vi "Tom_Bentham_New_FF.vi"() -> (5 "Plug in titles":string[](array[string]), 7 "Plug in values":string[](array[string]))   [LabVIEW 2010]
uses:
  Globals/Plug_in_data_global.vi
  Globals/Meas_global.vi
panel:
  out "max value":dbl format="%.2f"
  out "min value":dbl format="%.2f"
  out "FF":cluster{"Histogram of X":dbl[], "Axis":dbl[]}(graph)
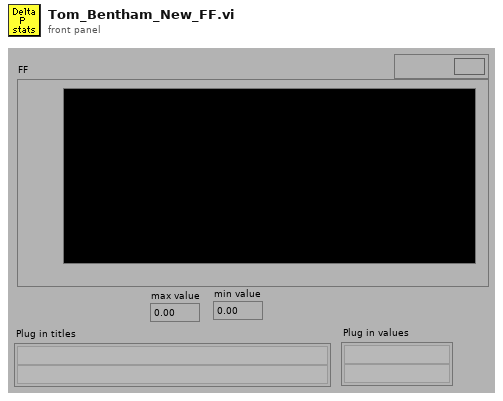
[diagram p1: front panel]
types:
  T1 = enum16{"Save no data", "Save data in new files", "Save data in existing files"}
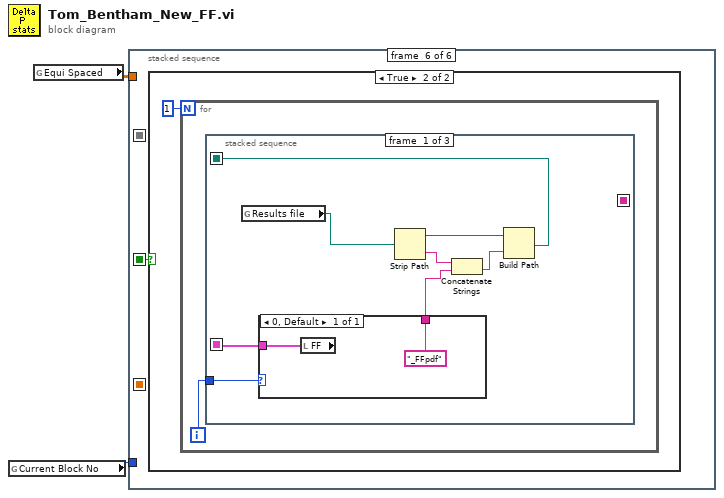
[diagram p0: block diagram]
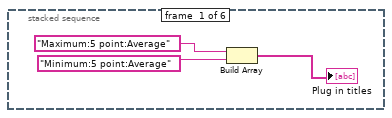
[diagram p2: hidden frame]
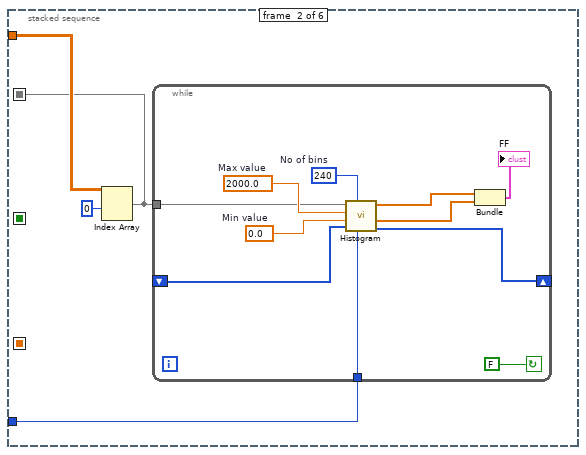
[diagram p3: hidden frame]
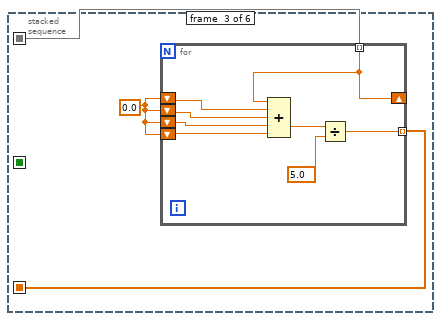
[diagram p4: hidden frame]
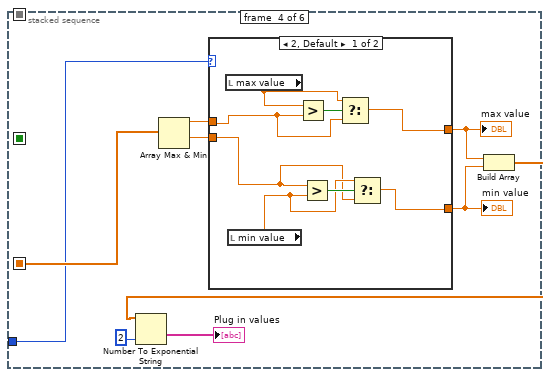
[diagram p5: hidden frame]
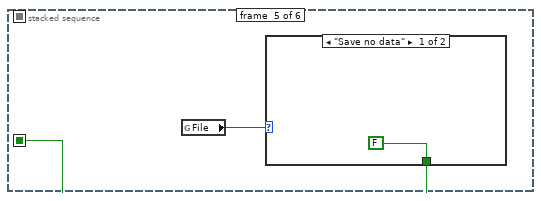
[diagram p7: hidden frame]
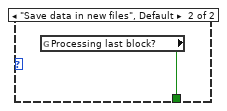
[diagram p8: hidden frame]
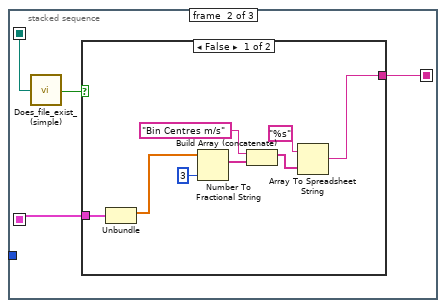
[diagram p10: hidden frame]
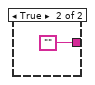
[diagram p11: hidden frame]
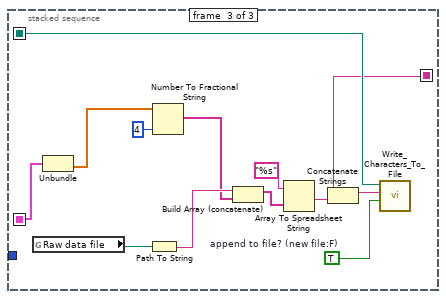
[diagram p12: hidden frame]
diagram:
  n1 = global read "Meas_global.vi" "Current Block No"() -> (w1:i32)
  n2 = global read "Plug_in_data_global.vi" "Equi Spaced"() -> (w2:dbl[][])
  n3 = stacked-sequence {
    seq-local: [_ w6 _ _ _ _] -> [_ _ w22 _ _ _]
    seq-local: [_ _ _ _ w51 _] -> [_ _ _ _ _ w55]
    seq-local: [_ _ w21 _ _ _] -> [_ _ _ w36 _ _]
    tunnel: w2 -> [_ w7 _ _ _ _]
    tunnel: w1 -> [_ w9 _ w35 _ _]
    frame #0 {
      n4 = Build Array("Maximum:5 point:Average", "Minimum:5 point:Average") -> (→"Plug in titles":string[])
    }
    frame #1 {
      n5 = Index Array(array=w7, index (row)=0) -> (element=w6:dbl[])  [unwired: 1 in]
      n6 = while {
        tunnel: w6 -> [w14]
        tunnel: w9 -> [w16]
        shift-left: _ -> [w15]
        shift-right: [w19] -> _
        stop <- FALSE continue-if-true
        w17 = 2000.0  # Max value
        w18 = 0.0  # Min value
        w20 = 240  # No of bins
        n7 = call "Histogram.vi"("Current Block No"=w16, "No of bins"=w20, "Shift Hist"=w15, "Min value"=w18, "Max value"=w17, "X"=w14) -> ("Shift Hist"=w19:i32[], "Histogram of X"=w12:dbl[], "Axis"=w13:dbl[])  [unwired: 2 in]
        n8 = Bundle("Axis"=w13, "Histogram of X"=w12) -> (→"FF":cluster{"Axis":dbl[], "Histogram of X":dbl[]})  [unwired: 1 in]
      }
    }
    frame #2 {
      w23 = 0.0
      n9 = for {
        shift-right: [w27] -> _
        shift-left: w23 -> [w31]
        shift-left: w23 -> [w30]
        shift-left: w23 -> [w29]
        shift-left: w23 -> [w28]
        tunnel: w22 -> [w27] mode=indexing
        tunnel: [w24] -> w21 mode=indexing
        n10 = Compound Arithmetic op=ADD(w27, w31, w30, w29, w28) -> (w26:dbl)
        n11 = Divide(x=w26, y=5.0) -> (x/y=w24:dbl)
      }
    }
    frame #3 {
      n12 = Array Max & Min(array=w36) -> (max value=w37:dbl, min value=w38:dbl)  [unwired: 2 out]
      n13 = case shown="2, Default" w35 {
        tunnel: [w45 w50] -> w39
        tunnel: w37 -> [w46 w50]
        tunnel: [w41 w49] -> w40
        tunnel: w38 -> [w42 w49]
        frame 2, Default {
          n14 = local read "max value"() -> (w47:dbl)
          n15 = local read "min value"() -> (w43:dbl)
          n16 = Greater?(x=w47, y=w46) -> (0:w48:bool)
          n17 = Greater?(x=w42, y=w43) -> (0:w44:bool)
          n18 = Select(t=w47, s=w48, f=w46) -> (s? t:f=w45:dbl)
          n19 = Select(t=w43, s=w44, f=w42) -> (s? t:f=w41:dbl)
        }
        frame 1 {
        }
      }
      "min value" <- w40
      "max value" <- w39
      n20 = Build Array(w39, w40) -> (w33:dbl[])
      n21 = Number To Exponential String(number=w33, precision (6)=2) -> (E-format string=→"Plug in values":string[])  [unwired: 2 in]
    }
    frame #4 {
      n22 = global read "Meas_global.vi" "File"() -> (w52:T1)
      n23 = case shown="\"Save no data\"" w52 {
        tunnel: [FALSE w54] -> w51
        frame "Save no data" {
        }
        frame "Save data in new files", Default {
          n24 = global read "Meas_global.vi" "Processing last block?"() -> (w54:bool)
        }
      }
    }
    frame #5 {
      n25 = case shown="True" w55 {
        frame False {
        }
        frame True {
          n26 = for {
            N: 1 -> [_]
            i -> [w57]
            n27 = stacked-sequence {
              seq-local: [w60 _ _] -> [_ w69 w86]
              seq-local: [w59 _ _] -> [_ w71 w85]
              seq-local: [_ w68 _] -> [_ _ w82]
              tunnel: w57 -> [w62 _ _]
              frame #0 {
                n28 = global read "Meas_global.vi" "Results file"() -> (w58:path)
                n29 = case shown="0, Default" w62 {
                  tunnel: ["_FFpdf" ("Substring")] -> w61
                  tunnel: [w66] -> w60
                  frame 0, Default {
                    n30 = local read "FF"() -> (w66:cluster{"Histogram of X":dbl[], "Axis":dbl[]})
                  }
                }
                n31 = Strip Path(path=w58) -> (stripped path=w65:path, name=w64:string)
                n32 = Concatenate Strings(w64, w61) -> (w63:string)
                n33 = Build Path(base path=w65, name or relative path=w63) -> (appended path=w59:path)
              }
              frame #1 {
                n34 = call "Does_file_exist_(simple).vi"("Pathname"=w71) -> ("exists?"=w70:bool)
                n35 = case shown="False" w70 {
                  tunnel: w69 -> [w79 _]
                  tunnel: [w72 ""] -> w68
                  frame False {
                    n36 = Unbundle(w79) -> ("Histogram of X"=w77:dbl[])  [unwired: 1 out]
                    n37 = Number To Fractional String(number=w77, precision (6)=i16 3) -> (F-format string=w74:string[])  [unwired: 2 in]
                    n38 = Build Array (concatenate)("Bin Centres m/s" ("Input Element"), w74) -> (w76:string[])
                    n39 = Array To Spreadsheet String(array=w76, 3:"%s" ("format string")) -> (spreadsheet string=w72:string)  [unwired: 1 in]
                  }
                  frame True {
                  }
                }
              }
              frame #2 {
                w87 = TRUE  # append to file? (new file:F)
                n40 = global read "Meas_global.vi" "Raw data file"() -> (w92:path)
                n41 = Unbundle(w86) -> ("Axis"=w84:dbl[])  [unwired: 1 out]
                n42 = Path To String(path=w92) -> (string=w91:string)
                n43 = Number To Fractional String(number=w84, precision (6)=i16 4) -> (F-format string=w90:string[])  [unwired: 2 in]
                n44 = Build Array (concatenate)(w91, w90) -> (w89:string[])
                n45 = Array To Spreadsheet String(array=w89, 3:"%s" ("format string")) -> (spreadsheet string=w83:string)  [unwired: 1 in]
                n46 = Concatenate Strings(w82, w83) -> (w81:string)
                n47 = call "Write_Characters_To_File.vi"("file path (dialog if empty)"=w85, "character string"=w81, "append to file? (new file:F)"=w87) -> ()  [unwired: 5 in, 1 out]
              }
            }
          }
        }
      }
    }
  }
